vi "HXG2_Write Cooling Htng.vi"(7 "Comp Contactor ON?":bool, 8 "error in (no error)":errorcluster, 11 "Alarm Cluster":T1) -> (0 "error out":errorcluster)   [LabVIEW 2012]
doc: "This VI will write outputs to the Digital Output card to energize compressor contactor, Air blower, Air heater, Gly pump, Gly htr contactor, Hot gas soln & Suct cool soln."
uses:
  Controls/HXG2_AlarmCluster.ctl
  Controls/UI/HXG2_LED.ctl
  Modules/EnableAirGly/HXG2enable.ctl
  Modules/DAQ/HXG2daq.ctl
  Controls/HXG2_DigitalOut.ctl
  <vilib>/DAQmx/write.llb/DAQmx Write (Digital 1D Bool NChan 1Samp 1Line).vi
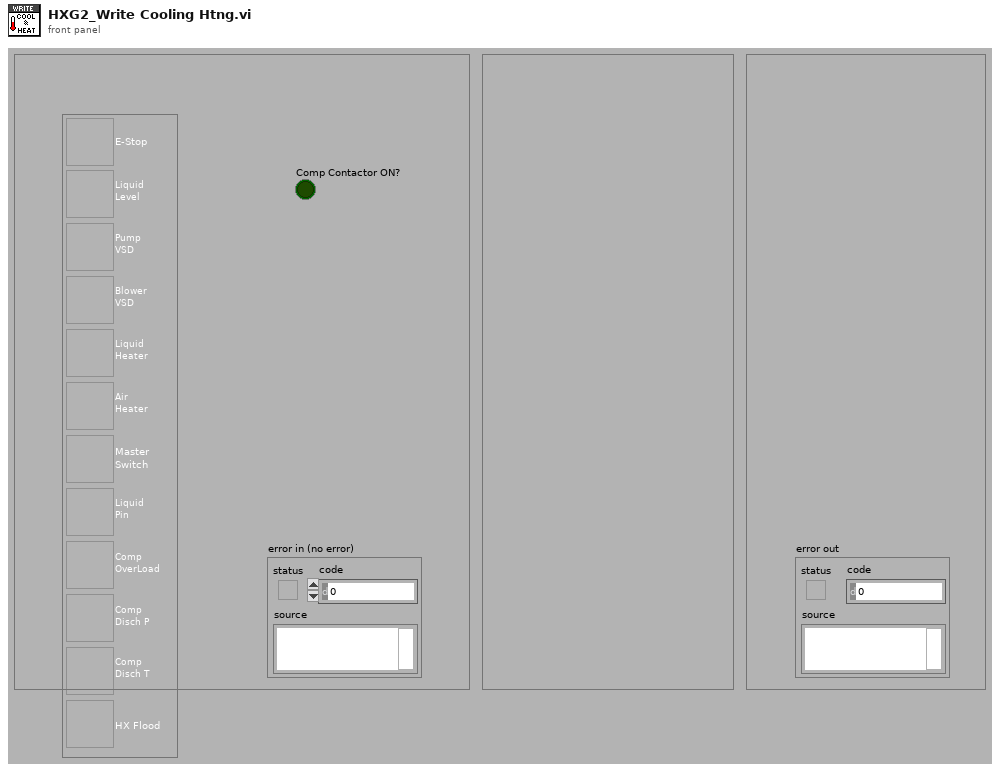
[diagram p1: front panel]
types:
  T1 = typedef "HXG2_AlarmCluster.ctl" = cluster{"E-Stop":T2, "Liquid\nLevel":T2, "Pump\nVSD":T2, "Blower\nVSD":T2, "Liquid\nHeater":T2, "Air\nHeater":T2, "Master\nSwitch":T2, "Liquid\nPin":T2, "Comp\nOverLoad":T2, "Comp\nDisch P":T2, "Comp \nDisch T":T2, "HX Flood":T2}
  T2 = typedef "HXG2_LED.ctl" = bool
  T3 = typedef "HXG2daq.ctl" = enum16{"Write", "Pass", "Initialize", "Stop"}
  T4 = typedef "HXG2enable.ctl" = enum16{"Write Refs", "Write", "Pass"}
  T5 = typedef "HXG2_DigitalOut.ctl" = cluster{"AirBlowerRUN":bool, "GlyPumpRUN":bool, "AirHtrCON":bool, "GlyHtrCON":bool, "CompCON":bool, "HotGasSoln":bool, "SuctCoolSoln":bool}
  T6 = cluster{"Air-Liq Out[0]":bool, "Air-Liq Out[1]":bool}
  T7 = typedef "HXG2_MaxConstants.ctl" = cluster{"IN":cluster{"all Digital":refnum<k21>, "all DAQ":refnum<k21>, "Analog 480panel":refnum<k21>, "Freq_Mdot":refnum<k21>}, "OUT":cluster{"DIGITAL":cluster{"all DIGITAL":refnum<k21>}, "allANALOG":cluster{"all ANALOG":refnum<k21>}}}
  T8 = cluster{"Air-Liq Refs[0]":refnum<vi>, "Air-Liq Refs[1]":refnum<vi>}
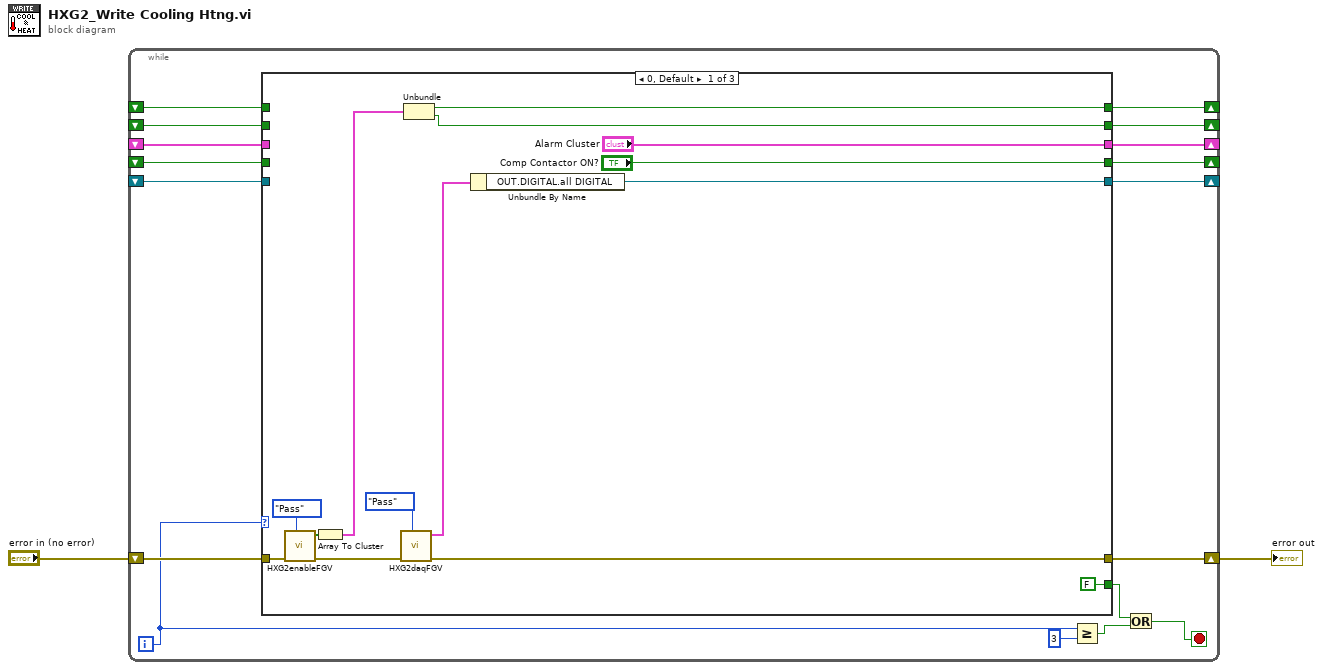
[diagram p0: block diagram]
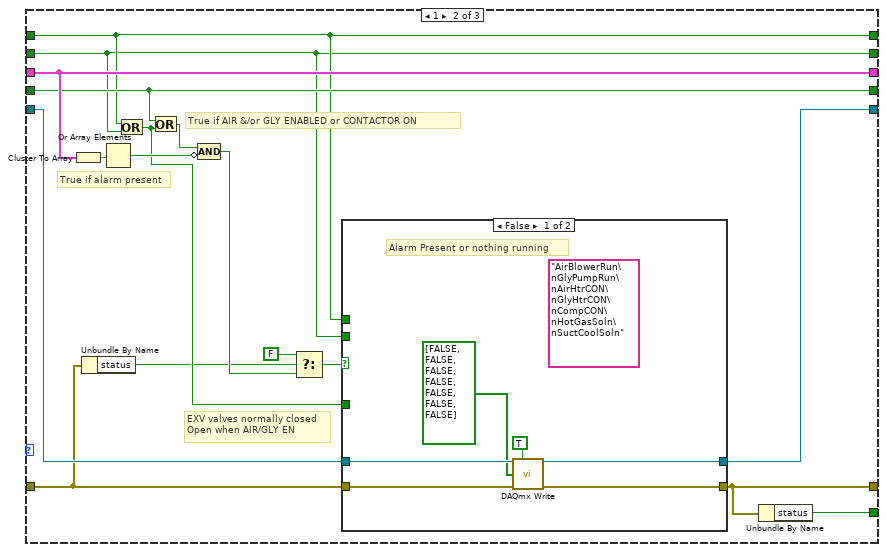
[diagram p2: hidden frame]
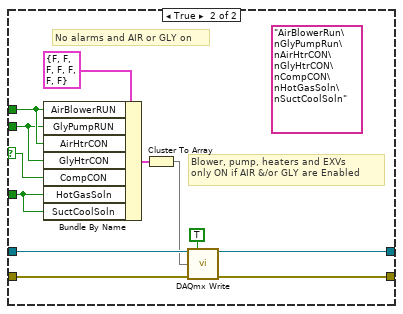
[diagram p3: hidden frame]
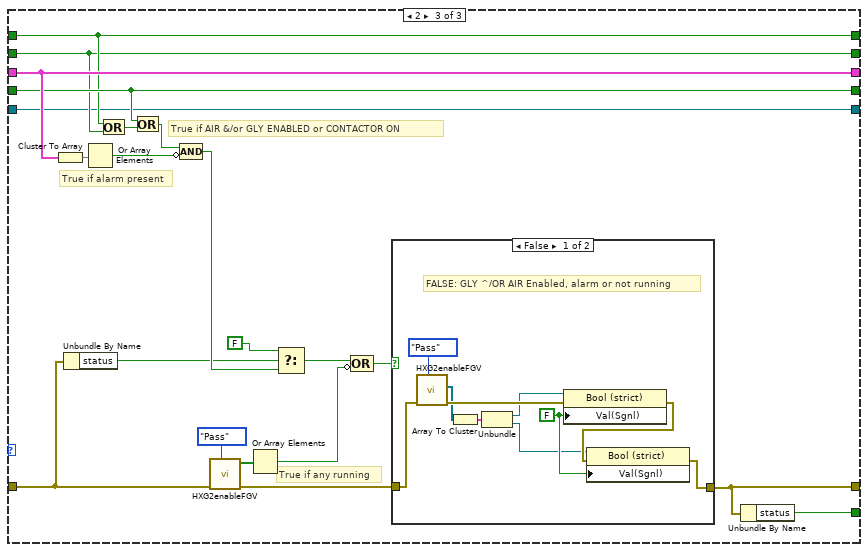
[diagram p4: hidden frame]
diagram:
  n1 = while {
    shift-right: [w19] -> _
    shift-left: _ -> [w17]
    shift-right: [w18] -> _
    shift-left: _ -> [w16]
    shift-right: [w15] -> _
    shift-left: _ -> [w14]
    shift-right: [w6] -> _
    shift-left: _ -> [w5]
    shift-right: [w4] -> _
    shift-left: _ -> [w3]
    shift-right: [w12] -> w1
    shift-left: "error in (no error)" -> [w13]
    i -> [w8]
    stop <- w9 stop-if-true
    n2 = case shown="0, Default" w8 {
      tunnel: [w28 w40 w84] -> w19
      tunnel: [w27 w39 w83] -> w18
      tunnel: w17 -> [_ w40 w84]
      tunnel: w16 -> [_ w39 w83]
      tunnel: ["Alarm Cluster" w48 w87] -> w15
      tunnel: w14 -> [_ w48 w87]
      tunnel: w13 -> [w29 w37 w78]
      tunnel: [w21 w44 w75] -> w12
      tunnel: [FALSE ("status") w50 w89] -> w11
      tunnel: ["Comp Contactor ON?" w46 w85] -> w6
      tunnel: w5 -> [_ w46 w85]
      tunnel: [w23 w42 w80] -> w4
      tunnel: w3 -> [_ w43 w80]
      frame 0, Default {
        n3 = call "HXG2enableFGV.vi"("ENABLE Ctrl"=HXG2enable."Pass" ("ENABLE"), "error in (no error)"=w29) -> ("error out"=w26:errorcluster, "Air-Liq Out"=w32:bool[])  [unwired: 7 in, 1 out]
        n4 = Array To Cluster(array=w32) -> (cluster=w31:T6)
        n5 = call "HXG2daqFGV.vi"("daqFGV"=HXG2daq."Pass", "error in (no error)"=w26) -> ("error out"=w21:errorcluster, "MAX"=w24:T7)  [unwired: 8 in]
        n6 = Unbundle(w31) -> ("Air-Liq Out[0]"=w28:bool, "Air-Liq Out[1]"=w27:bool)
        n7 = Unbundle By Name(w24) -> ("OUT.DIGITAL.all DIGITAL"=w23:refnum<k21>)
      }
      frame 1 {
        # "EXV valves normally closed\nOpen when AIR/GLY EN"
        # "True if alarm present"
        # "True if AIR &/or GLY ENABLED or CONTACTOR ON"
        n8 = Cluster To Array(cluster=w48) -> (array=w49:T2[])
        n9 = Unbundle By Name(w37) -> ("status"=w36:bool)
        n10 = Or Array Elements(Boolean array=w49) -> (logical OR=w47:bool)
        n11 = Or(x=w40, y=w39) -> (x .or. y?=w41:bool)
        n12 = Or(x=w46, y=w41) -> (x .or. y?=w45:bool)
        n13 = Compound Arithmetic op=AND(w45, invert w47) -> (w38:bool)
        n14 = Select(t=FALSE, s=w36, f=w38) -> (s? t:f=w35:bool)
        n15 = case shown="False" w35 {
          selector: w35 -> [_ w59]
          tunnel: w37 -> [w54 w68]
          tunnel: [w55 w67] -> w44
          tunnel: w43 -> [w56 w65]
          tunnel: [w52 w64] -> w42
          tunnel: w41 -> [_ w60]
          tunnel: w40 -> [_ w58]
          tunnel: w39 -> [_ w57]
          frame False {
            (unwired) "AirBlowerRun\nGlyPumpRun\nAirHtrCON\nGlyHtrCON\nCompCON\nHotGasSoln\nSuctCoolSoln"
            # "Alarm Present or nothing running"
            n16 = call-poly <vilib>:"DAQmx Write.vi"("task/channels in"=w56, "auto start"=TRUE, "data"=bool[] [FALSE, FALSE, FALSE, FALSE, FALSE, FALSE, FALSE], "error in"=w54) -> ("task out"=w52:refnum<k21>, "error out"=w55:errorcluster)  [unwired: 9 in, 1 out]
          }
          frame True {
            (unwired) "AirBlowerRun\nGlyPumpRun\nAirHtrCON\nGlyHtrCON\nCompCON\nHotGasSoln\nSuctCoolSoln"
            # "Blower, pump, heaters and EXVs\nonly ON if AIR &/or GLY are Enabled"
            # "No alarms and AIR or GLY on"
            n17 = Bundle By Name(cluster=T5 {"AirBlowerRUN"=FALSE, "GlyPumpRUN"=FALSE, "AirHtrCON"=FALSE, "GlyHtrCON"=FALSE, "CompCON"=FALSE, "HotGasSoln"=FALSE, "SuctCoolSoln"=FALSE} ("DigitalOut"), "AirBlowerRUN"=w58, "GlyPumpRUN"=w57, "AirHtrCON"=w58, "GlyHtrCON"=w57, "CompCON"=w59, "HotGasSoln"=w60, "SuctCoolSoln"=w60) -> (w62:T5)
            n18 = Cluster To Array(cluster=w62) -> (array=w61:bool[])
            n19 = call-poly <vilib>:"DAQmx Write.vi"("task/channels in"=w65, "auto start"=TRUE, "data"=w61, "error in"=w68) -> ("task out"=w64:refnum<k21>, "error out"=w67:errorcluster)  [unwired: 9 in, 1 out]
          }
        }
        n20 = Unbundle By Name(w44) -> ("status"=w50:bool)
      }
      frame 2 {
        # "True if AIR &/or GLY ENABLED or CONTACTOR ON"
        # "True if any running"
        # "True if alarm present"
        n21 = Cluster To Array(cluster=w87) -> (array=w88:T2[])
        n22 = Unbundle By Name(w78) -> ("status"=w81:bool)
        n23 = Or Array Elements(Boolean array=w88) -> (logical OR=w86:bool)
        n24 = Or(x=w84, y=w83) -> (x .or. y?=w70:bool)
        n25 = Or(x=w85, y=w70) -> (x .or. y?=w71:bool)
        n26 = Compound Arithmetic op=AND(w71, invert w86) -> (w82:bool)
        n27 = call "HXG2enableFGV.vi"("ENABLE Ctrl"=HXG2enable."Pass" ("ENABLE"), "error in (no error)"=w78) -> ("error out"=w76:errorcluster, "Air-Liq Out"=w77:bool[])  [unwired: 7 in, 1 out]
        n28 = Or Array Elements(Boolean array=w77) -> (logical OR=w72:bool)
        n29 = Select(t=FALSE, s=w81, f=w82) -> (s? t:f=w73:bool)
        n30 = Compound Arithmetic op=OR(w73, invert w72) -> (w74:bool)
        n31 = case shown="False" w74 {
          tunnel: w76 -> [w99 w100]
          tunnel: [w95 w100] -> w75
          frame False {
            w94 = FALSE ("Value (Signaling)")
            # "FALSE: GLY ^/OR AIR Enabled, alarm or not running"
            n32 = call "HXG2enableFGV.vi"("ENABLE Ctrl"=HXG2enable."Pass" ("ENABLE"), "error in (no error)"=w99) -> ("error out"=w97:errorcluster, "Air-Liq Refs"=w93:refnum<vi>[])  [unwired: 7 in, 1 out]
            n33 = Array To Cluster(array=w93) -> (cluster=w92:T8)
            n34 = Unbundle(w92) -> ("Air-Liq Refs[0]"=w91:refnum<vi>, "Air-Liq Refs[1]"=w90:refnum<vi>)
            n35 = property class="Bool (strict)"(reference=w91, error in=w97, "Val(Sgnl)"=w94) -> (error out=w96:errorcluster)  [unwired: 1 out]
            n36 = property class="Bool (strict)"(reference=w90, error in=w96, "Val(Sgnl)"=w94) -> (error out=w95:errorcluster)  [unwired: 1 out]
          }
          frame True {
          }
        }
        n37 = Unbundle By Name(w75) -> ("status"=w89:bool)
      }
    }
    n38 = Greater Or Equal?(x=w8, y=3) -> (x >= y?=w10:bool)
    n39 = Or(x=w11, y=w10) -> (x .or. y?=w9:bool)
  }
  "error out" <- w1
